vi "MTMount_getSample_General.vi"(8 "error in (no error)":errorcluster, 11 "General_Ctl":T1) -> (0 "error out":errorcluster, 2 "function return":i32, 3 "General_Ctl out":T1)   [LabVIEW 2018, in "SALLV_MTMount.lvlib"]
doc: "int MTMount_shm_getSample_GeneralLV(MTMount_GeneralLV *General_Ctl );"
uses:
  SALLV_MTMount.lvlib
  DataTypes/General.ctl
  SALLV_MTMount.so
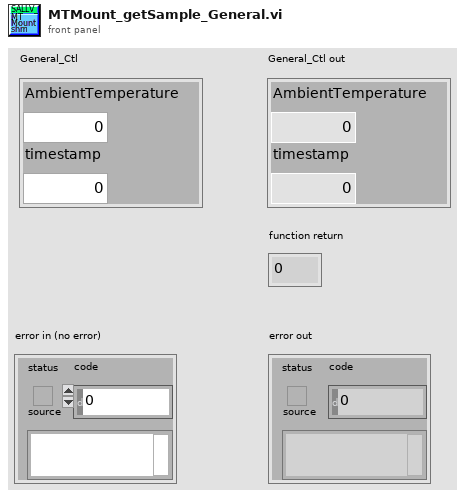
[diagram p1: front panel]
types:
  T1 = typedef "SALLV_MTMount.lvlib/General.ctl" = cluster{"AmbientTemperature":dbl, "timestamp":dbl}
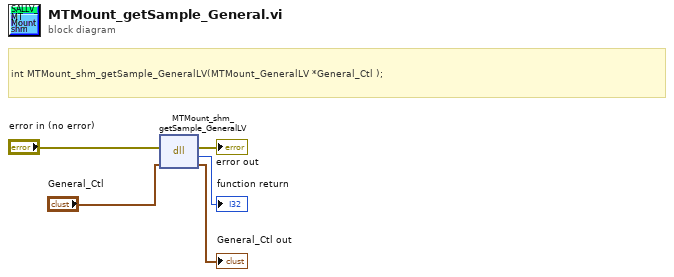
[diagram p0: block diagram]
diagram:
  # "int MTMount_shm_getSample_GeneralLV(MTMount_GeneralLV *General_Ctl );"
  n1 = dll-call lib="home/ttsai/Document/salApiMTMount/SALLV_MTMount/SALLV_MTMount.*" fn="MTMount_shm_getSample_GeneralLV"(error in="error in (no error)", "General_Ctl"="General_Ctl") -> (error out=→"error out":errorcluster, →"function return":i32, "General_Ctl"=→"General_Ctl out":T1)  [unwired: 2 in, 1 out]
